vi "mainWTControl.vi"() -> ()   [LabVIEW 2017]
panel:
  out "Density":dbl
  out "Wind Velocity":dbl
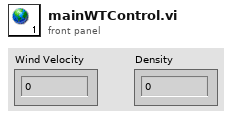
[diagram p1: front panel]
diagram:
